vi "FRCts20_Backend_XMLBenchmark.vi"() -> ()   [LabVIEW 2014, in "FRCts20_Backend_TestCode.lvlib"]
uses:
  FRCts20_Backend_TestCode.lvlib
  FRCts20_Backend_IssueDfn.ctl
  FRCts20_Backend_Controls.lvlib
  FRCts20_Backend_TeamDfn.ctl
  FRCts20_Backend_TeamDataDfn.ctl
  FRCts20_Backend_request_info.ctl
  FRCts20_Backend_Note.ctl
  FRCts20_Backend_Note_list.ctl
  FRCts20_Backend_IssueTeamList.ctl
  FRCts20_Backend_Team_Info.ctl
panel:
  in  "data 4":T1
  in  "Path":path=path "C:/FRC Team Service/source/Static Source/FRCts20_Backend_XMLMain.xml"
  out "data 3":T1
  in  "error in (no error) 3":errorcluster
  out "error out 3":errorcluster
  out "Total Parse Time":u32
  in  "XML String In":string
  out "XML String":string
  out "error out 2":errorcluster
  out "Total Gen Time":u32
  in  "error in (no error) 2":errorcluster
  out "Total Open Time":u32
  out "error out":errorcluster
  in  "error in (no error)":errorcluster
  out "data":T1
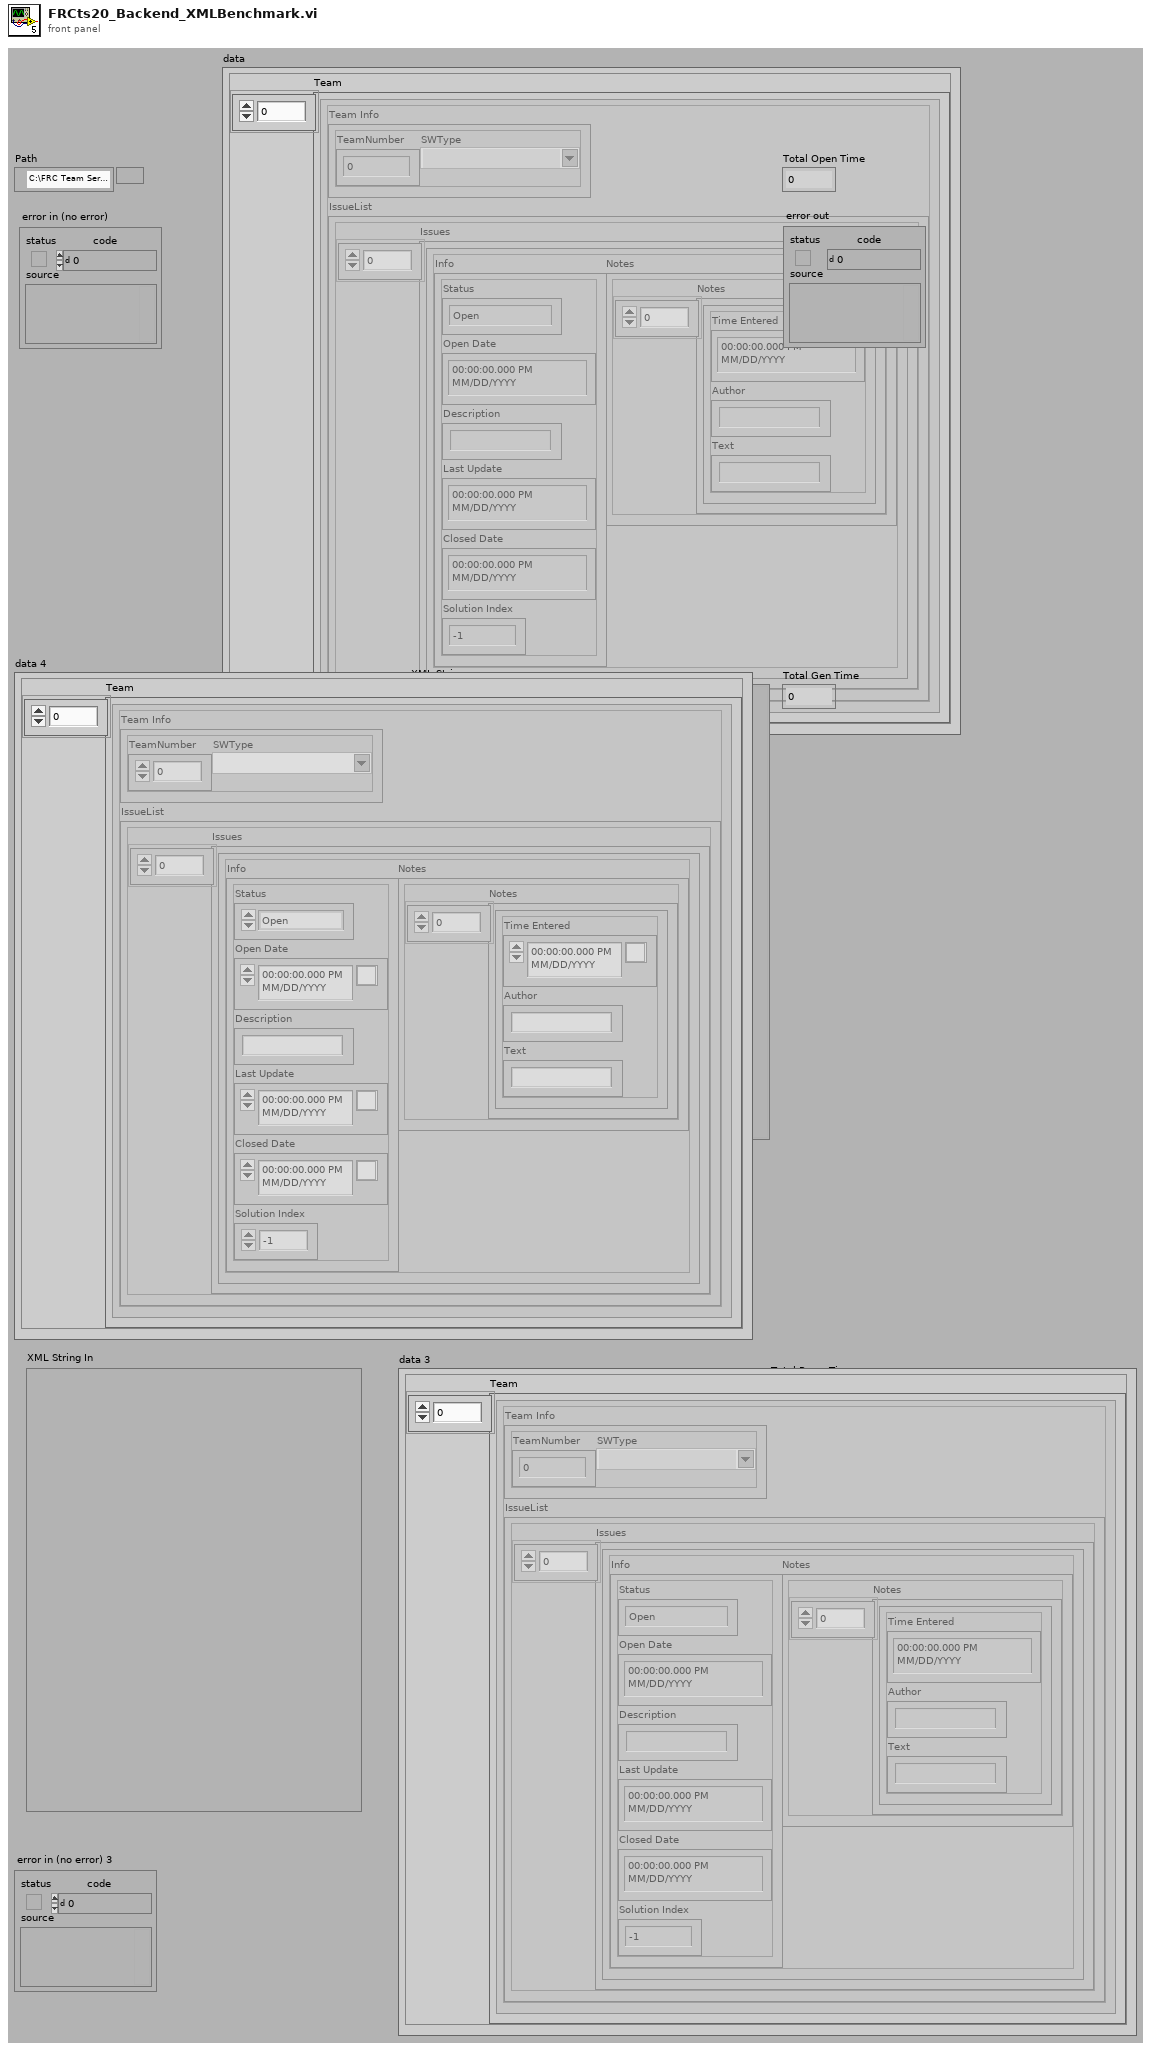
[diagram p1: front panel]
types:
  T1 = typedef "FRCts20_Backend_Controls.lvlib/FRCts20_Backend_TeamDataDfn.ctl" = cluster{"Team":T2[]}
  T2 = typedef "FRCts20_Backend_Controls.lvlib/FRCts20_Backend_TeamDfn.ctl" = cluster{"Team Info":T3, "IssueList":T4}
  T3 = typedef "FRCts20_Backend_Controls.lvlib/FRCts20_Backend_Team_Info.ctl" = cluster{"TeamNumber":u16, "SWType":string}
  T4 = typedef "FRCts20_Backend_Controls.lvlib/FRCts20_Backend_IssueTeamList.ctl" = cluster{"Issues":T5[]}
  T5 = typedef "FRCts20_Backend_Controls.lvlib/FRCts20_Backend_IssueDfn.ctl" = cluster{"Notes":T6, "Info":T8}
  T6 = typedef "FRCts20_Backend_Controls.lvlib/FRCts20_Backend_Note_list.ctl" = cluster{"Notes":T7[]}
  T7 = typedef "FRCts20_Backend_Controls.lvlib/FRCts20_Backend_Note.ctl" = cluster{"Time Entered":timestamp, "Author":string, "Text":string}
  T8 = typedef "FRCts20_Backend_Controls.lvlib/FRCts20_Backend_request_info.ctl" = cluster{"Status":enum16{"Open", "In Work", "Closed"}, "Open Date":timestamp, "Description":string, "Last Update":timestamp, "Closed Date":timestamp, "Solution Index":i32}
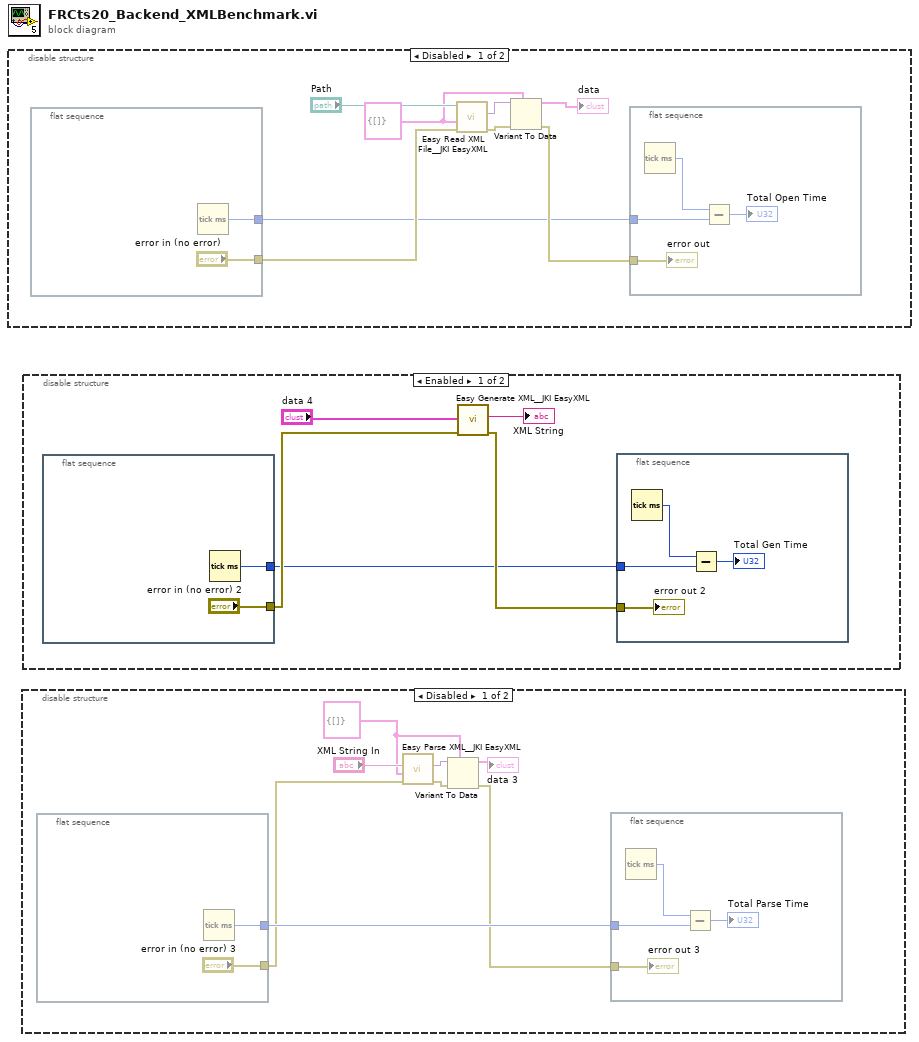
[diagram p0: block diagram]
diagram:
  n1 = disable-structure shown="Disabled" {
    frame Disabled {
      w6 = T1 {"Team"=[]} ("TeamData")
      n2 = flat-sequence {
        tunnel: ["error in (no error)"] -> w3
        tunnel: [w13] -> w1
        frame #0 {
          n3 = Tick Count (ms)() -> (millisecond timer value=w13:u32)
        }
      }
      n4 = call <vilib>:"Easy Read XML File__JKI EasyXML.vi"("error in (no error)"=w3, "LabVIEW Data (Type)"=w6, "XML File Path"="Path") -> ("error out"=w7:errorcluster, "LabVIEW Data"=w5:variant)  [unwired: 6 in, 1 out]
      n5 = Variant To Data(error in=w7, type=w6, Variant=w5) -> (data=→"data":T1, error out=w2:errorcluster)
      n6 = flat-sequence {
        tunnel: w2 -> [w12]
        tunnel: w1 -> [w10]
        frame #0 {
          n7 = Tick Count (ms)() -> (millisecond timer value=w11:u32)
          n8 = Subtract(x=w11, y=w10) -> (x-y=→"Total Open Time":u32)
          "error out" <- w12
        }
      }
    }
    frame Enabled {
    }
  }
  n9 = disable-structure shown="Disabled" {
    frame Disabled {
      w16 = T1 {"Team"=[]} ("TeamData")
      n10 = flat-sequence {
        tunnel: ["error in (no error) 3"] -> w20
        tunnel: [w27] -> w21
        frame #0 {
          n11 = Tick Count (ms)() -> (millisecond timer value=w27:u32)
        }
      }
      n12 = call <vilib>:"Easy Parse XML__JKI EasyXML.vi"("error in (no error)"=w20, "LabVIEW Data (Type)"=w16, "XML String"="XML String In") -> ("error out"=w19:errorcluster, "LabVIEW Data"=w17:variant)  [unwired: 7 in]
      n13 = Variant To Data(error in=w19, type=w16, Variant=w17) -> (data=→"data 3":T1, error out=w18:errorcluster)
      n14 = flat-sequence {
        tunnel: w18 -> [w26]
        tunnel: w21 -> [w24]
        frame #0 {
          n15 = Tick Count (ms)() -> (millisecond timer value=w25:u32)
          n16 = Subtract(x=w25, y=w24) -> (x-y=→"Total Parse Time":u32)
          "error out 3" <- w26
        }
      }
    }
    frame Enabled {
    }
  }
  n17 = disable-structure shown="Enabled" {
    frame Enabled {
      n18 = flat-sequence {
        tunnel: ["error in (no error) 2"] -> w33
        tunnel: [w38] -> w31
        frame #0 {
          n19 = Tick Count (ms)() -> (millisecond timer value=w38:u32)
        }
      }
      n20 = call <vilib>:"Easy Generate XML__JKI EasyXML.vi"("error in (no error)"=w33, "LabVIEW Data"="data 4") -> ("error out"=w32:errorcluster, "XML String"=→"XML String":string)  [unwired: 8 in]
      n21 = flat-sequence {
        tunnel: w32 -> [w37]
        tunnel: w31 -> [w35]
        frame #0 {
          n22 = Tick Count (ms)() -> (millisecond timer value=w36:u32)
          n23 = Subtract(x=w36, y=w35) -> (x-y=→"Total Gen Time":u32)
          "error out 2" <- w37
        }
      }
    }
    frame Disabled {
    }
  }
